vi "L41.vi"() -> ()   [LabVIEW 2014]
panel:
  in  "L41":dbl
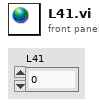
[diagram p1: front panel]
diagram:
